vi "启动.vi"   [LabVIEW 2015]
uses:
  <vilib>/ActorFramework/Actor/Actor.lvclass
  <vilib>/Instr/_visa.llb/VISA Configure Serial Port (Instr).vi
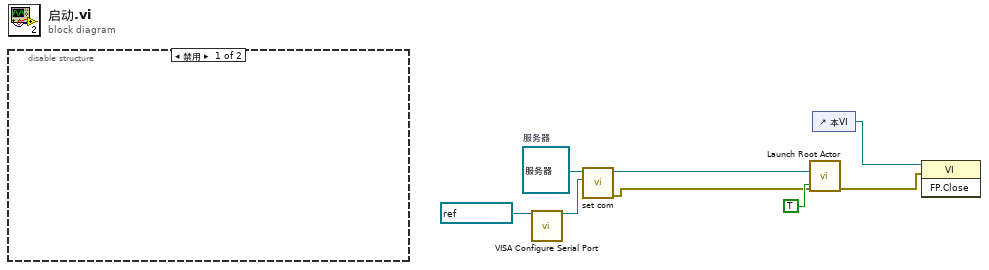
[diagram p0: block diagram]
diagram:
  w8 = refnum<class "服务器.lvclass"> refnum  # 服务器
  n1 = disable-structure shown="禁用" {
    frame Disabled {
    }
    frame Enabled {
    }
  }
  n2 = call-poly "VISA Configure Serial Port"("VISA resource name"=refnum<visa-resource-name> "COM30") -> ("VISA resource name out"=w7:refnum<visa-resource-name>)  [unwired: 13 in, 1 out]
  n3 = call "set com.vi"("COM"=w7, "串口参数管理 输入"=w8) -> ("error out"=w3:errorcluster, "串口参数管理 输出"=w4:refnum<class "服务器.lvclass">)  [unwired: 8 in]
  n4 = call <vilib>:"Launch Root Actor.vi"("Open Actor Core front panel? (F)"=TRUE, "error in (no error)"=w3, "Actor"=w4) -> ("error out"=w2:errorcluster)  [unwired: 7 in, 1 out]
  n5 = control-ref of="本VI"() -> (w1:refnum<vi>)
  n6 = invoke class="VI" method="FP.Close"(reference=w1, error in=w2) -> ()  [unwired: 1 in, 3 out]
